vi "Resampling a Waveform (single-shot).vi"() -> ()   [LabVIEW 2020]
doc: "This example demonstrates the effect of resampling a waveform in single-shot mode and the impact of the different resampling parameters. Single-shot mode is used when resampling a single block of the signal. Continuous mode is used when resampling separate but contiguous blocks of the signal."
uses:
  <vilib>/measure/maresamp.llb/Resample Waveform (single shot).vi
  <vilib>/Waveform/WDTOps.llb/WDT Number of Waveform Samples DBL.vi
  <vilib>/measure/NI_MAPro.lvlib
panel:
  out "Number of Resampled Samples":i32
  in  "Stop":bool
  out "Original and Resampled Waveforms":waveform(dbl)[](graph)
  in  "Output Rate (Hz)":dbl=5500.0
  in  "t0":dbl(slide) scale=-0.002..0.002
  # "Overview: Demonstrates the effect of resampling a waveform in single-shot mode.\nRequirements: LabVIEW Full Development System\nInstructions:\n1. Run the VI. Observe the difference between the Input Waveform and the Resampled Waveform.\n2. Change the values of t0 and Output Rate and observe the change in the graph.\n3. Click Stop to stop the VI."
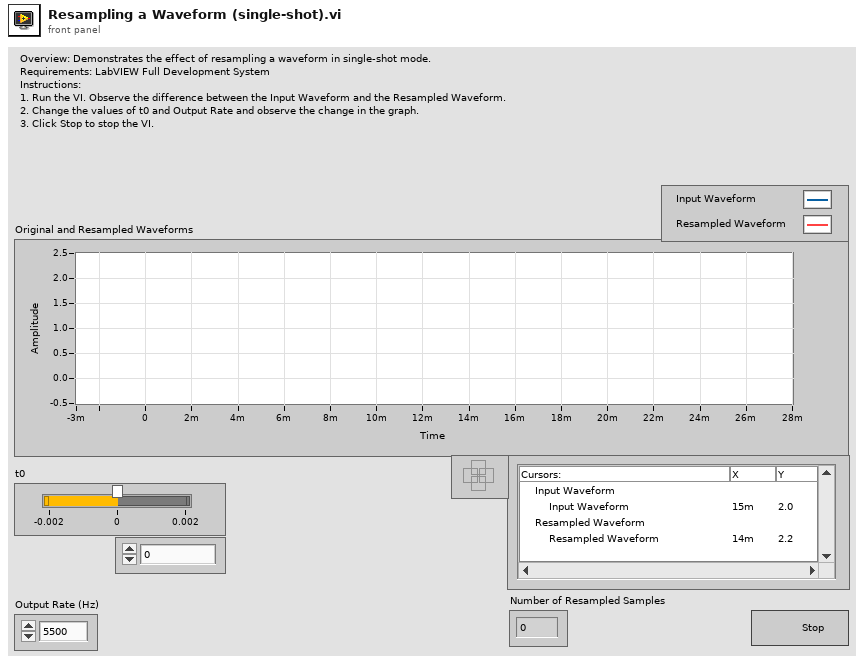
[diagram p1: front panel]
types:
  T1 = cluster{"alias rejection (dB)":dbl, "normalized bandwidth":dbl}
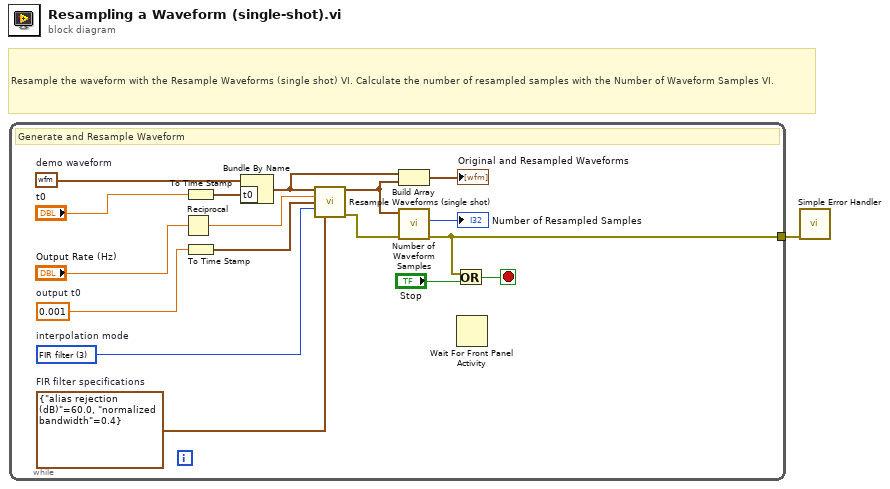
[diagram p0: block diagram]
diagram:
  # "Resample the waveform with the Resample Waveforms (single shot) VI. Calculate the number of resampled samples with the Number of Waveform Samples VI."
  n1 = while {
    tunnel: [w2] -> w1
    stop <- w3 stop-if-true
    w11 = waveform(dbl) {"t0"=timestamp(0 s since 1904-01-01), "dt"=0.001, "Y"=[0.0, 0.5, 1.5, 2.0, 1.5, 0.5000000000000002, 0.0, 0.4999999999999998, 1.4999999999999998, 2.0, 2.0, 2.0, 2.0, 2.0, 2.0, 2.0, 0.0, 0.0, 0.0, 0.0, 1.0, 0.0, 0.0, 0.0, 0.0]}  # demo waveform
    w6 = 0.001  # output t0
    w8 = T1 {"alias rejection (dB)"=60.0, "normalized bandwidth"=0.4}  # FIR filter specifications
    w9 = u16 3 items=["coerce", "linear", "spline", "FIR filter"]  # interpolation mode
    # "Generate and Resample Waveform"
    n2 = Reciprocal(x="Output Rate (Hz)") -> (1/x=w12:dbl)
    n3 = To Time Stamp(1:"t0") -> (0:w7:timestamp)
    n4 = To Time Stamp(1:w6) -> (0:w5:timestamp)
    n5 = Bundle By Name(cluster=w11, "t0"=w7) -> (w16:waveform(dbl))
    n6 = call-poly <vilib>:"Resample Waveforms (single shot).vi"("waveform in"=w16, "dt"=w12, "t0"=w5, "interpolation mode"=w9, "FIR filter specifications"=w8) -> ("resampled waveform out"=w14:waveform(dbl), "error out"=w4:errorcluster)  [unwired: 2 in, 7 out]
    n7 = Build Array(w16, w14) -> (→"Original and Resampled Waveforms":waveform(dbl)[])
    n8 = call-poly <vilib>:"Number of Waveform Samples.vi"("error in (no error)"=w4, "waveform in"=w14) -> ("error out"=w2:errorcluster, "number of samples"=→"Number of Resampled Samples":i32)  [unwired: 8 out]
    n9 = Or(x=w2, y="Stop") -> (x .or. y?=w3:bool)
    n10 = Wait For Front Panel Activity() -> ()  [unwired: 3 in, 1 out]
  }
  n11 = call <vilib>:"Simple Error Handler.vi"("error in (no error)"=w1) -> ()  [unwired: 4 in, 5 out]
